vi "Parse Git Flow Config.vi"(11 "standard output":string="Branch name for production releases: master \nBranch name for \"next release\" development: develop \nFeature branch prefix: feature/ \nBugfix branch prefix: bugfix/ \nRelease branch prefix: release/ \nHotfix branch prefix: hotfix/ \nSupport branch prefix: support/ \nVersion tag prefix:  \n") -> (3 "Array":cluster{"key":string, "value":string}[](array[cluster]))   [LabVIEW 2019, in "Git.lvclass"]
uses:
  Git.lvclass
panel:
  out "Array 2":string[][](array[string])
  out "Git FLow Branches":T1
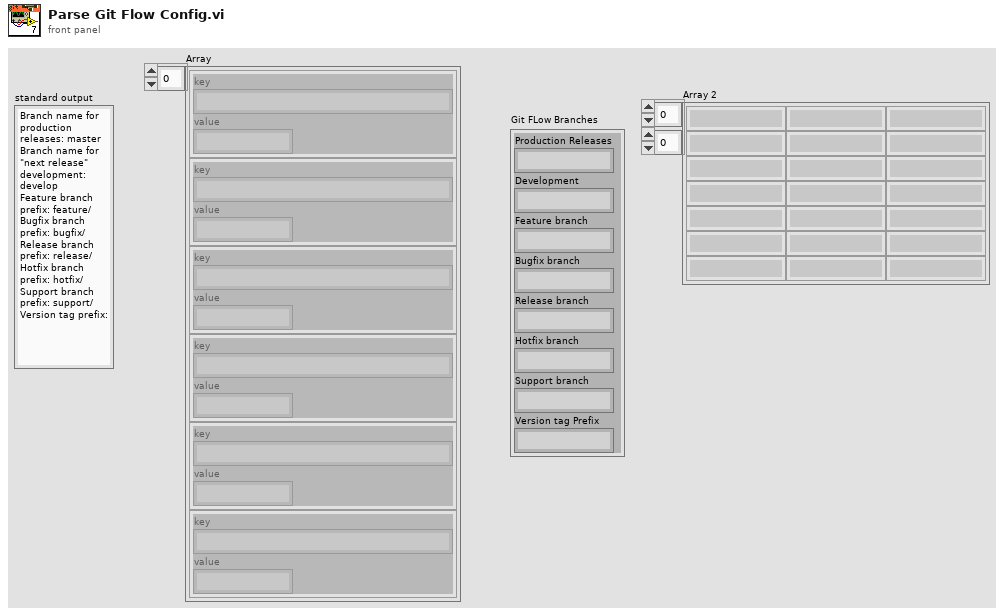
[diagram p1: front panel]
types:
  T1 = cluster{"Production Releases":string, "Development":string, "Feature branch":string, "Bugfix branch":string, "Release branch":string, "Hotfix branch":string, "Support branch":string, "Version tag Prefix":string}
  T2 = cluster{"Production Release":string, "Development":string, "Feature Prefix":string, "Bugfix Prefix":string, "Release Prefix":string, "Hotfix Prefix":string, "Support Prefix":string, "Version tag Prefix":string}
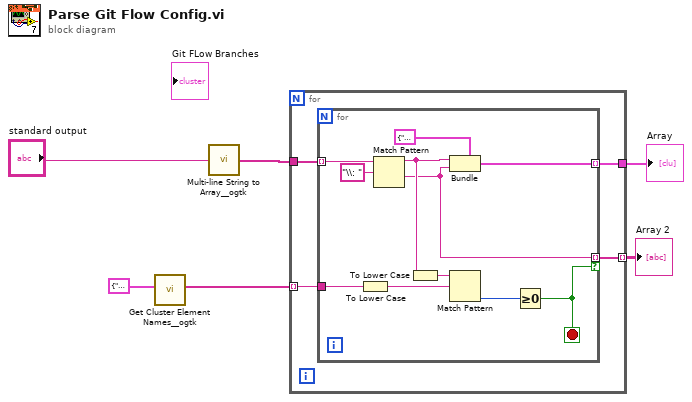
[diagram p0: block diagram]
diagram:
  n1 = call <userlib>:"Get Cluster Element Names__ogtk.vi"("Cluster"=T2 {"Production Release"="master ", "Development"="master ", "Feature Prefix"="master ", "Bugfix Prefix"="master ", "Release Prefix"="master ", "Hotfix Prefix"="master ", "Support Prefix"="master ", "Version tag Prefix"="master "} ("Git FLow Branches")) -> ("Element Names"=w2:string[])  [unwired: 9 in, 1 out]
  n2 = call <userlib>:"Multi-line String to Array__ogtk.vi"("string"="standard output") -> ("lines"=w5:string[])
  n3 = for {
    tunnel: w5 -> [w10]
    tunnel: [w9] -> w4
    tunnel: w2 -> [w8] mode=indexing
    tunnel: [w7] -> w1 mode=indexing
    n4 = for {
      tunnel: w10 -> [w20] mode=indexing
      tunnel: [w19] -> w9 mode=indexing
      tunnel: w8 -> [w17]
      tunnel: [w14] -> w7 mode=indexing if=w13
      stop <- w13 stop-if-true
      n5 = To Lower Case(string=w17) -> (all lower case string=w11:string)
      n6 = Match Pattern(string=w20, regular expression="\\: ") -> (before substring=w15:string, after substring=w14:string)  [unwired: 1 in, 2 out]
      n7 = To Lower Case(string=w15) -> (all lower case string=w12:string)
      n8 = Bundle(cluster=cluster{"key":string, "value":string} {"key"="", "value"=""} ("key-value"), "key"=w15, "value"=w14) -> (w19:cluster{"key":string, "value":string})
      n9 = Match Pattern(string=w12, regular expression=w11) -> (offset past match=w16:i32)  [unwired: 1 in, 3 out]
      n10 = Greater Or Equal To 0?(x=w16) -> (x >= 0?=w13:bool)
    }
  }
  "Array" <- w4
  "Array 2" <- w1
